vi "Track boiler with Pixy.vi"() -> (0 "%error":dbl, 1 "sees boiler":bool, 2 "y output":dbl, 3 "x output":dbl)   [LabVIEW 2016]
uses:
  Robot Global Data.vi
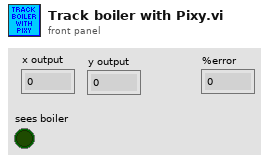
[diagram p1: front panel]
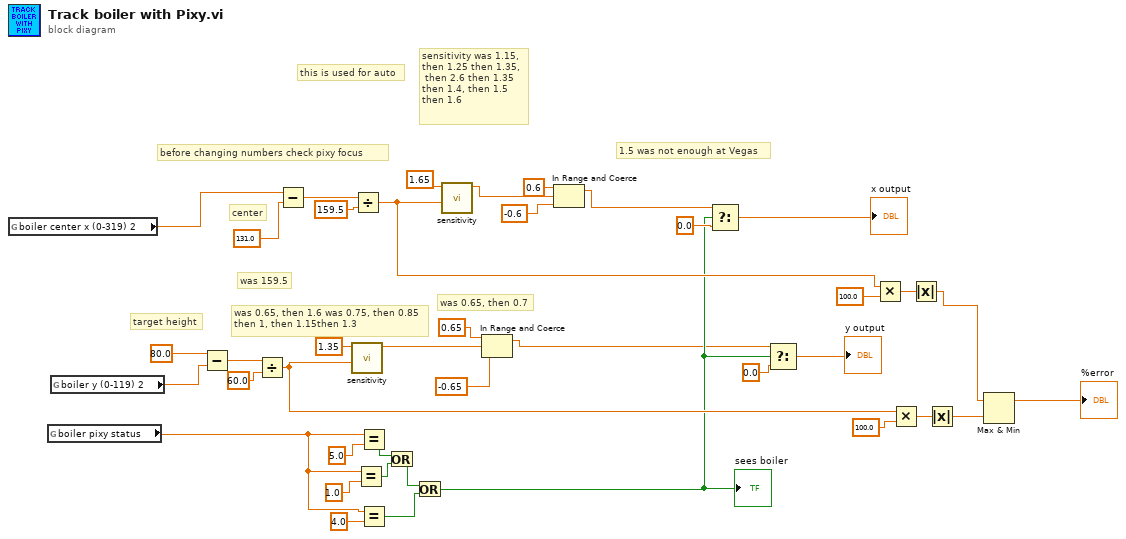
[diagram p0: block diagram]
diagram:
  # "was 0.65, then 0.7"
  # "was 159.5"
  # "was 0.65, then 1.6 was 0.75, then 0.85\nthen 1, then 1.15then 1.3"
  # "1.5 was not enough at Vegas"
  # "sensitivity was 1.15, \nthen 1.25 then 1.35,\n then 2.6 then 1.35 \nthen 1.4, then 1.5\nthen 1.6"
  # "center"
  # "target height"
  # "this is used for auto"
  # "before changing numbers check pixy focus"
  n1 = global read "Robot Global Data.vi" "boiler center x (0-319) 2"() -> (w36:dbl)
  n2 = global read "Robot Global Data.vi" "boiler pixy status"() -> (w29:dbl)
  n3 = global read "Robot Global Data.vi" "boiler y (0-119) 2"() -> (w9:dbl)
  n4 = Subtract(x=80.0 ("y"), y=w9) -> (x-y=w25:dbl)
  n5 = Divide(x=w25, y=60.0) -> (x/y=w22:dbl)
  n6 = Subtract(x=w36, y=131.0) -> (x-y=w39:dbl)
  n7 = call "sensitivity.vi"("x"=w22, "sensitivity"=1.35) -> ("scaled value"=w8:dbl)  [unwired: 9 in]
  n8 = Divide(x=w39, y=159.5) -> (x/y=w14:dbl)
  n9 = Equal?(x=w29, y=1.0) -> (x = y?=w31:bool)
  n10 = Equal?(x=w29, y=5.0) -> (x = y?=w32:bool)
  n11 = Equal?(x=w29, y=4.0) -> (x = y?=w27:bool)
  n12 = Or(x=w32, y=w31) -> (x .or. y?=w26:bool)
  n13 = Or(x=w26, y=w27) -> (x .or. y?=w11:bool)
  "sees boiler" <- w11
  n14 = call "sensitivity.vi"("x"=w14, "sensitivity"=1.65) -> ("scaled value"=w4:dbl)  [unwired: 9 in]
  n15 = In Range and Coerce(upper limit=0.65, x=w8, lower limit=-0.65) -> (coerced(x)=w7:dbl)  [unwired: 1 out]
  n16 = In Range and Coerce(upper limit=0.6, x=w4, lower limit=-0.6) -> (coerced(x)=w3:dbl)  [unwired: 1 out]
  n17 = Select(t=w3, s=w11, f=0.0) -> (s? t:f=→"x output":dbl)
  n18 = Select(t=w7, s=w11, f=0.0) -> (s? t:f=→"y output":dbl)
  n19 = Multiply(x=w14, y=100.0) -> (x*y=w16:dbl)
  n20 = Multiply(x=w22, y=100.0) -> (x*y=w20:dbl)
  n21 = Absolute Value(x=w16) -> (abs(x)=w15:dbl)
  n22 = Absolute Value(x=w20) -> (abs(x)=w19:dbl)
  n23 = Max & Min(x=w15, y=w19) -> (max(x,y)=→"%error":dbl)  [unwired: 1 out]
